vi "stop.vi"(8 "error in (no error)":errorcluster, 11 "TestResult in":refnum<class "TestResult.lvclass">) -> (0 "error out":errorcluster, 3 "TestResult out":refnum<class "TestResult.lvclass">)   [LabVIEW 2011, in "TestResult.lvclass"]
uses:
  TestResult.lvclass
  private/shouldStop.ctl
  TestResult.lvclass/TestResult.ctl
panel:
  # "JKI VI Tester for LabVIEW\nhttp://jkisoft.com/vi-tester\nCopyright (C) 2007-2009, JKI <info@jkisoft.com>\nALL RIGHTS RESERVED"
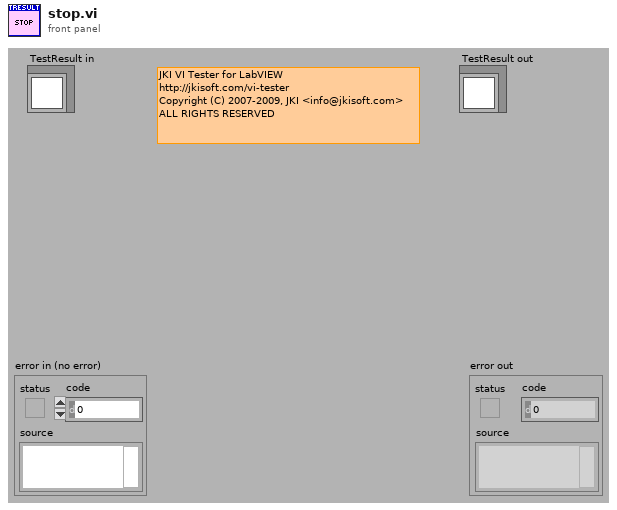
[diagram p1: front panel]
types:
  T1 = typedef "TestResult.lvclass/shouldStop.ctl" = bool
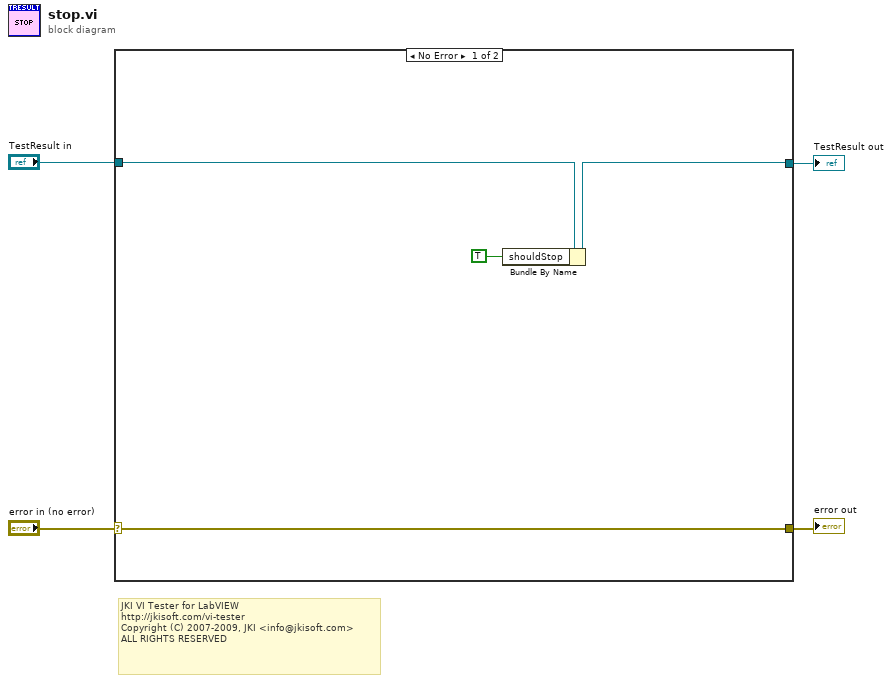
[diagram p0: block diagram]
diagram:
  # "JKI VI Tester for LabVIEW\nhttp://jkisoft.com/vi-tester\nCopyright (C) 2007-2009, JKI <info@jkisoft.com>\nALL RIGHTS RESERVED"
  n1 = case shown="No Error" "error in (no error)" {
    selector: "error in (no error)" -> [w8 w10]
    tunnel: [w8 w10] -> w3
    tunnel: [w6 w9] -> w1
    tunnel: "TestResult in" -> [w7 w9]
    frame No Error {
      n2 = Bundle By Name(cluster=w7, "shouldStop"=T1 TRUE) -> (w6:refnum<class "TestResult.lvclass">)
    }
    frame Error {
    }
  }
  "error out" <- w3
  "TestResult out" <- w1
